vi "Is Concrete Class.vi"(0 "Vector Path Group in":refnum<class "Vector Path Group.lvclass">, 11 "error in (no error)":errorcluster) -> (4 "Vector Path Group out":refnum<class "Vector Path Group.lvclass">, 6 "Is Concrete Class?":bool=TRUE, 15 "error out":errorcluster)   [LabVIEW 2023, in "RFFixtureCharact.Public.lvlib" / "Vector Path Group.lvclass"]
uses:
  Vector Path Group.lvclass
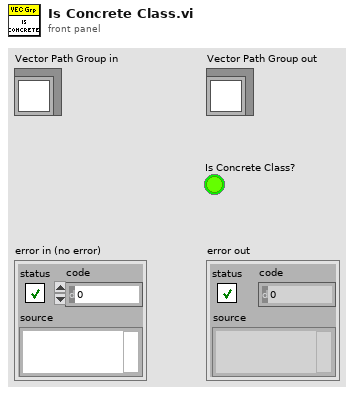
[diagram p1: front panel]
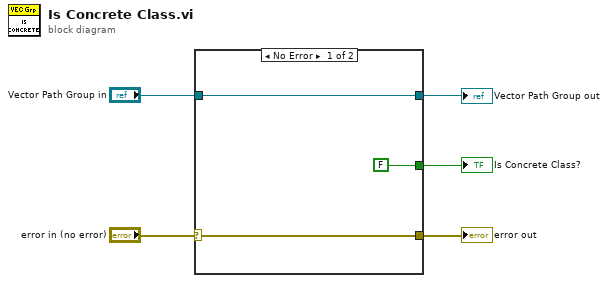
[diagram p0: block diagram]
diagram:
  n1 = case shown="No Error" "error in (no error)" {
    selector: "error in (no error)" -> [w7 w10]
    tunnel: [FALSE ("Is Concrete Class?") _] -> w2
    tunnel: [w7 w10] -> w1
    tunnel: [w6 w9] -> w3
    tunnel: "Vector Path Group in" -> [w6 w9]
    frame No Error {
    }
    frame Error {
    }
  }
  "error out" <- w1
  "Vector Path Group out" <- w3
  "Is Concrete Class?" <- w2
